vi "Result_Test.vi"(8 "error in (no error)":errorcluster caption="entrée d'erreur (pas d'erreur)", 11 "Get_Voltage en entrée":refnum<class "Read_Multimeter_Voltage.lvclass">) -> (0 "error out":errorcluster caption="sortie d'erreur", 3 "Get_Voltage en sortie":refnum<class "Read_Multimeter_Voltage.lvclass">)   [LabVIEW 2020, in "Library Test.lvlib" / "Read_Multimeter_Voltage.lvclass"]
uses:
  Read_Multimeter_Voltage.lvclass
  C:/Users/ngarcin/OneDrive - Altyor/Standard TB/Suite TB45/Class/Test/Test (Default)/Test (Default).lvclass
  Commun VI/TypeDef/Variable Printable.ctl
  Read_Multimeter.lvclass
  Commun VI/Library Commun.lvlib
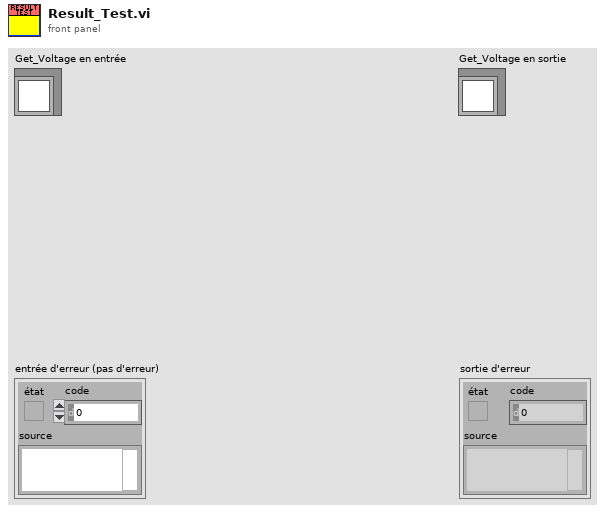
[diagram p1: front panel]
types:
  T1 = typedef "Variable Printable.ctl" = string
  T2 = enum16{"Get Variable", "Get All Variables", "Set Variable", "Delete Variable", "Delete All Variable"}
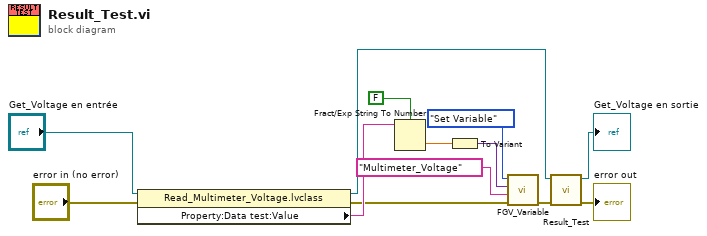
[diagram p0: block diagram]
diagram:
  n1 = property class="Read_Multimeter_Voltage.lvclass"(reference="Get_Voltage en entrée", error in="error in (no error)") -> (reference out=w5:refnum<class "Read_Multimeter_Voltage.lvclass">, error out=w4:errorcluster, "Property:Data test:Value"=w11:string)
  n2 = Fract/Exp String To Number(use system decimal point (T)=FALSE ("utiliser le séparateur décimal du système (V)"), string=w11) -> (number=w2:dbl)  [unwired: 2 in, 1 out]
  n3 = To Variant(anything=w2) -> (Variant=w8:variant)
  n4 = call "FGV_Variable.vi"("error in (no error)"=w4, "Variable"=T1 "Multimeter_Voltage", "Data In"=w8, "Function"=T2."Set Variable") -> ("error out"=w3:errorcluster)  [unwired: 5 in, 2 out]
  n5 = call-parent "Result_Test.vi"("error in (no error)"=w3, "Get_Voltage en entrée"=w5) -> ("error out"=→"error out":errorcluster, "Get_Voltage en sortie"=→"Get_Voltage en sortie":refnum<class "Read_Multimeter_Voltage.lvclass">)  [unwired: 8 in]
